vi "nanocal -- nuclear schottky fit V8.vi"() -> ()   [LabVIEW 2021] (continued)
\"σlogτS\" -> 0.000000000000   ,  \"σlogτN\" -> 0.000000000000   ,  \"σητ1\" -> 0.000000000000   ,  \"σητS \" -> 0.000000000000   ,  \"σητN\" -> 0.000000000000    |>   , \n\"IDS0571_220607_RAW_cal__ref_\" ->   <|    \"ζ\" -> 0.017026202892   ,  \"τ1\" -> 0.018855414009   ,  \"τS\" -> 0.047086117348   ,  \"τN\" -> 0.000023679327   ,  \"τC\" -> 0.002651600111   ,  \"κ0\" -> 0.000000012631   ,  \"mm1\" -> 0.000042096925   ,  \"mm2\" -> 0.018841082396   ,  \"mm3\" -> 0.050535732431   ,  \"T\" -> 1.900000000000   ,  \"B\" -> 2.000000000000   ,  \"θ\" -> 0.000000000000   ,  \"Reoff\" -> -457142.857142857042   ,  \"Imoff\" -> 0.000000000000   ,  \"στ1\" -> 0.700233981740   ,  \"στS\" -> 0.000265032226   ,  \"στN\" -> 0.457232881356   ,  \"τ11 \" -> 0.000000000000   ,  \"τ12\" -> 0.000000000000   ,  \"τ22\" -> 0.000000000000   ,  \"τN1\" -> 0.000000000000   ,  \"τN2\" -> 0.000000000000   ,  \"σηlogτ1 \" -> 0.000000000000   ,  \"σηlogτS\" -> 0.000000000000   ,  \"σηlogτN\" -> 0.000000000000   ,  \"σlogτ1\" -> 0.000000000000   ,  \"σlogτS\" -> 0.000000000000   ,  \"σlogτN\" -> 0.000000000000   ,  \"σητ1\" -> 0.000000000000   ,  \"σητS \" -> 0.000000000000   ,  \"σητN\" -> 0.000000000000    |>   , \n\"IDS0571_220607_RAW_cal__sam_\" ->   <|    \"ζ\" -> 0.000000000000   ,  \"τ1\" -> 0.000000000000   ,  \"τS\" -> 0.000000000000   ,  \"τN\" -> 0.000000000000   ,  \"τC\" -> 0.000000000000   ,  \"κ0\" -> 0.000000000000   ,  \"mm1\" -> 0.000000000000   ,  \"mm2\" -> 0.000000000000   ,  \"mm3\" -> 0.000000000000   ,  \"T\" -> 1.900000000000   ,  \"B\" -> 2.000000000000   ,  \"θ\" -> 0.000000000000   ,  \"Reoff\" -> 0.000000000000   ,  \"Imoff\" -> 0.000000000000   ,  \"στ1\" -> 0.000000000000   ,  \"στS\" -> 0.000000000000   ,  \"στN\" -> 0.000000000000   ,  \"τ11 \" -> 0.000000000000   ,  \"τ12\" -> 0.000000000000   ,  \"τ22\" -> 0.000000000000   ,  \"τN1\" -> 0.000000000000   ,  \"τN2\" -> 0.000000000000   ,  \"σηlogτ1 \" -> 0.000000000000   ,  \"σηlogτS\" -> 0.000000000000   ,  \"σηlogτN\" -> 0.000000000000   ,  \"σlogτ1\" -> 0.000000000000   ,  \"σlogτS\" -> 0.000000000000   ,  \"σlogτN\" -> 0.000000000000   ,  \"σητ1\" -> 0.000000000000   ,  \"σητS \" -> 0.000000000000   ,  \"σητN\" -> 0.000000000000    |>   , \n\"IDS0572_220607_RAW_cal__ref_\" ->   <|    \"ζ\" -> 0.018157472970   ,  \"τ1\" -> 0.020617918401   ,  \"τS\" -> 0.014016495736   ,  \"τN\" -> 0.000014742683   ,  \"τC\" -> 0.002574156451   ,  \"κ0\" -> 0.000000016091   ,  \"mm1\" -> 0.000038981702   ,  \"mm2\" -> 0.016741377131   ,  \"mm3\" -> 0.020697726271   ,  \"T\" -> 2.300000000000   ,  \"B\" -> 2.000000000000   ,  \"θ\" -> 0.000000000000   ,  \"Reoff\" -> -420408.163265306036   ,  \"Imoff\" -> 0.000000000000   ,  \"στ1\" -> 0.362521056079   ,  \"στS\" -> 0.000160694817   ,  \"στN\" -> 0.168025207283   ,  \"τ11 \" -> 0.000000000000   ,  \"τ12\" -> 0.000000000000   ,  \"τ22\" -> 0.000000000000   ,  \"τN1\" -> 0.000000000000   ,  \"τN2\" -> 0.000000000000   ,  \"σηlogτ1 \" -> 0.000000000000   ,  \"σηlogτS\" -> 0.000000000000   ,  \"σηlogτN\" -> 0.000000000000   ,  \"σlogτ1\" -> 0.000000000000   ,  \"σlogτS\" -> 0.000000000000   ,  \"σlogτN\" -> 0.000000000000   ,  \"σητ1\" -> 0.000000000000   ,  \"σητS \" -> 0.000000000000   ,  \"σητN\" -> 0.000000000000    |>   , \n\"IDS0572_220607_RAW_cal__sam_\" ->   <|    \"ζ\" -> 0.000000000000   ,  \"τ1\" -> 0.000000000000   ,  \"τS\" -> 0.000000000000   ,  \"τN\" -> 0.000000000000   ,  \"τC\" -> 0.000000000000   ,  \"κ0\" -> 0.000000000000   ,  \"mm1\" -> 0.000000000000   ,  \"mm2\" -> 0.000000000000   ,  \"mm3\" -> 0.000000000000   ,  \"T\" -> 2.300000000000   ,  \"B\" -> 2.000000000000   ,  \"θ\" -> 0.000000000000   ,  \"Reoff\" -> 0.000000000000   ,  \"Imoff\" -> 0.000000000000   ,  \"στ1\" -> 0.000000000000   ,  \"στS\" -> 0.000000000000   ,  \"στN\" -> 0.000000000000   ,  \"τ11 \" -> 0.000000000000   ,  \"τ12\" -> 0.000000000000   ,  \"τ22\" -> 0.000000000000   ,  \"τN1\" -> 0.000000000000   ,  \"τN2\" -> 0.000000000000   ,  \"σηlogτ1 \" -> 0.000000000000   ,  \"σηlogτS\" -> 0.000000000000   ,  \"σηlogτN\" -> 0.000000000000   ,  \"σlogτ1\" -> 0.000000000000   ,  \"σlogτS\" -> 0.000000000000   ,  \"σlogτN\" -> 0.000000000000   ,  \"σητ1\" -> 0.000000000000   ,  \"σητS \" -> 0.000000000000   ,  \"σητN\" -> 0.000000000000    |>   , \n\"IDS0573_220607_RAW_cal__ref_\" ->   <|    \"ζ\" -> 0.021415792037   ,  \"τ1\" -> 0.017082452868   ,  \"τS\" -> 0.009548586507   ,  \"τN\" -> 0.000007399205   ,  \"τC\" -> 0.002472586118   ,  \"κ0\" -> 0.000000022500   ,  \"mm1\" -> 0.000041498148   ,  \"mm2\" -> 0.012165481918   ,  \"mm3\" -> 0.017108693634   ,  \"T\" -> 3.100000000000   ,  \"B\" -> 2.000000000000   ,  \"θ\" -> 0.000000000000   ,  \"Reoff\" -> -261224.489795918343   ,  \"Imoff\" -> 0.000000000000   ,  \"στ1\" -> 0.720539777711   ,  \"στS\" -> 0.000216738961   ,  \"στN\" -> 0.337779672751   ,  \"τ11 \" -> 0.000000000000   ,  \"τ12\" -> 0.000000000000   ,  \"τ22\" -> 0.000000000000   ,  \"τN1\" -> 0.000000000000   ,  \"τN2\" -> 0.000000000000   ,  \"σηlogτ1 \" -> 0.000000000000   ,  \"σηlogτS\" -> 0.000000000000   ,  \"σηlogτN\" -> 0.000000000000   ,  \"σlogτ1\" -> 0.000000000000   ,  \"σlogτS\" -> 0.000000000000   ,  \"σlogτN\" -> 0.000000000000   ,  \"σητ1\" -> 0.000000000000   ,  \"σητS \" -> 0.000000000000   ,  \"σητN\" -> 0.000000000000    |>   , \n\"IDS0573_220607_RAW_cal__sam_\" ->   <|    \"ζ\" -> 0.000000000000   ,  \"τ1\" -> 0.000000000000   ,  \"τS\" -> 0.000000000000   ,  \"τN\" -> 0.000000000000   ,  \"τC\" -> 0.000000000000   ,  \"κ0\" -> 0.000000000000   ,  \"mm1\" -> 0.000000000000   ,  \"mm2\" -> 0.000000000000   ,  \"mm3\" -> 0.000000000000   ,  \"T\" -> 3.100000000000   ,  \"B\" -> 2.000000000000   ,  \"θ\" -> 0.000000000000   ,  \"Reoff\" -> 0.000000000000   ,  \"Imoff\" -> 0.000000000000   ,  \"στ1\" -> 0.000000000000   ,  \"στS\" -> 0.000000000000   ,  \"στN\" -> 0.000000000000   ,  \"τ11 \" -> 0.000000000000   ,  \"τ12\" -> 0.000000000000   ,  \"τ22\" -> 0.000000000000   ,  \"τN1\" -> 0.000000000000   ,  \"τN2\" -> 0.000000000000   ,  \"σηlogτ1 \" -> 0.000000000000   ,  \"σηlogτS\" -> 0.000000000000   ,  \"σηlogτN\" -> 0.000000000000   ,  \"σlogτ1\" -> 0.000000000000   ,  \"σlogτS\" -> 0.000000000000   ,  \"σlogτN\" -> 0.000000000000   ,  \"σητ1\" -> 0.000000000000   ,  \"σητS \" -> 0.000000000000   ,  \"σητN\" -> 0.000000000000    |>   , \n\"IDS0574_220607_RAW_cal__ref_\" ->   <|    \"ζ\" -> 0.022252360347   ,  \"τ1\" -> 0.015843819663   ,  \"τS\" -> 0.005763523322   ,  \"τN\" -> 0.000001375995   ,  \"τC\" -> 0.001974723590   ,  \"κ0\" -> 0.000000055533   ,  \"mm1\" -> 0.000032327889   ,  \"mm2\" -> 0.007832797575   ,  \"mm3\" -> 0.015846599723   ,  \"T\" -> 5.700000000000   ,  \"B\" -> 2.000000000000   ,  \"θ\" -> 0.000000000000   ,  \"Reoff\" -> -92244.897959183683   ,  \"Imoff\" -> 0.000000000000   ,  \"στ1\" -> 6.958139019645   ,  \"στS\" -> 0.000482683411   ,  \"στN\" -> 3.920374328535   ,  \"τ11 \" -> 0.000000000000   ,  \"τ12\" -> 0.000000000000   ,  \"τ22\" -> 0.000000000000   ,  \"τN1\" -> 0.000000000000   ,  \"τN2\" -> 0.000000000000   ,  \"σηlogτ1 \" -> 0.000000000000   ,  \"σηlogτS\" -> 0.000000000000   ,  \"σηlogτN\" -> 0.000000000000   ,  \"σlogτ1\" -> 0.000000000000   ,  \"σlogτS\" -> 0.000000000000   ,  \"σlogτN\" -> 0.000000000000   ,  \"σητ1\" -> 0.000000000000   ,  \"σητS \" -> 0.000000000000   ,  \"σητN\" -> 0.000000000000    |>   , \n\"IDS0574_220607_RAW_cal__sam_\" ->   <|    \"ζ\" -> 0.000000000000   ,  \"τ1\" -> 0.000000000000   ,  \"τS\" -> 0.000000000000   ,  \"τN\" -> 0.000000000000   ,  \"τC\" -> 0.000000000000   ,  \"κ0\" -> 0.000000000000   ,  \"mm1\" -> 0.000000000000   ,  \"mm2\" -> 0.000000000000   ,  \"mm3\" -> 0.000000000000   ,  \"T\" -> 5.700000000000   ,  \"B\" -> 2.000000000000   ,  \"θ\" -> 0.000000000000   ,  \"Reoff\" -> 0.000000000000   ,  \"Imoff\" -> 0.000000000000   ,  \"στ1\" -> 0.000000000000   ,  \"στS\" -> 0.000000000000   ,  \"στN\" -> 0.000000000000   ,  \"τ11 \" -> 0.000000000000   ,  \"τ12\" -> 0.000000000000   ,  \"τ22\" -> 0.000000000000   ,  \"τN1\" -> 0.000000000000   ,  \"τN2\" -> 0.000000000000   ,  \"σηlogτ1 \" -> 0.000000000000   ,  \"σηlogτS\" -> 0.000000000000   ,  \"σηlogτN\" -> 0.000000000000   ,  \"σlogτ1\" -> 0.000000000000   ,  \"σlogτS\" -> 0.000000000000   ,  \"σlogτN\" -> 0.000000000000   ,  \"σητ1\" -> 0.000000000000   ,  \"σητS \" -> 0.000000000000   ,  \"σητN\" -> 0.000000000000    |>   , \n\"IDS0578_220608_RAW_cal__ref_\" ->   <|    \"ζ\" -> 0.254942126755   ,  \"τ1\" -> 0.090194641149   ,  \"τS\" -> 0.019458727705   ,  \"τN\" -> 0.002319182302   ,  \"τC\" -> 0.000961097925   ,  \"κ0\" -> 0.000000000915   ,  \"mm1\" -> 0.000189263930   ,  \"mm2\" -> 0.024128719117   ,  \"mm3\" -> 0.094167772727   ,  \"T\" -> 0.200000000000   ,  \"B\" -> 2.000000000000   ,  \"θ\" -> 90.000000000000   ,  \"Reoff\" -> 0.000000000000   ,  \"Imoff\" -> 0.000000000000   ,  \"στ1\" -> 0.002629714713   ,  \"στS\" -> 0.000006197246   ,  \"στN\" -> 0.000056566732   ,  \"τ11 \" -> 0.000000000000   ,  \"τ12\" -> 0.000000000000   ,  \"τ22\" -> 0.000000000000   ,  \"τN1\" -> 0.000000000000   ,  \"τN2\" -> 0.000000000000   ,  \"σηlogτ1 \" -> 0.069428028467   ,  \"σηlogτS\" -> 0.000045157290   ,  \"σηlogτN\" -> 0.118005576339   ,  \"σlogτ1\" -> 0.029155997290   ,  \"σlogτS\" -> 0.000318481580   ,  \"σlogτN\" -> 0.024390808828   ,  \"σητ1\" -> 0.006262036113   ,  \"σητS \" -> 0.000000878703   ,  \"σητN\" -> 0.000273676444    |>   , \n\"IDS0578_220608_RAW_cal__sam_\" ->   <|    \"ζ\" -> 0.000000000000   ,  \"τ1\" -> 0.000000000000   ,  \"τS\" -> 0.000000000000   ,  \"τN\" -> 0.000000000000   ,  \"τC\" -> 0.000000000000   ,  \"κ0\" -> 0.000000000000   ,  \"mm1\" -> 0.000000000000   ,  \"mm2\" -> 0.000000000000   ,  \"mm3\" -> 0.000000000000   ,  \"T\" -> 0.200000000000   ,  \"B\" -> 2.000000000000   ,  \"θ\" -> 90.000000000000   ,  \"Reoff\" -> 0.000000000000   ,  \"Imoff\" -> 0.000000000000   ,  \"στ1\" -> 0.000000000000   ,  \"στS\" -> 0.000000000000   ,  \"στN\" -> 0.000000000000   ,  \"τ11 \" -> 0.000000000000   ,  \"τ12\" -> 0.000000000000   ,  \"τ22\" -> 0.000000000000   ,  \"τN1\" -> 0.000000000000   ,  \"τN2\" -> 0.000000000000   ,  \"σηlogτ1 \" -> 0.000000000000   ,  \"σηlogτS\" -> 0.000000000000   ,  \"σηlogτN\" -> 0.000000000000   ,  \"σlogτ1\" -> 0.000000000000   ,  \"σlogτS\" -> 0.000000000000   ,  \"σlogτN\" -> 0.000000000000   ,  \"σητ1\" -> 0.000000000000   ,  \"σητS \" -> 0.000000000000   ,  \"σητN\" -> 0.000000000000    |>   , \n\"IDS0579_220608_RAW_cal__ref_\" ->   <|    \"ζ\" -> 0.354589792209   ,  \"τ1\" -> 0.123845684439   ,  \"τS\" -> 0.022131661400   ,  \"τN\" -> 0.006759309931   ,  \"τC\" -> 0.000842117409   ,  \"κ0\" -> 0.000000000715   ,  \"mm1\" -> 0.000215927769   ,  \"mm2\" -> 0.027938681410   ,  \"mm3\" -> 0.135668607521   ,  \"T\" -> 0.170000000000   ,  \"B\" -> 2.000000000000   ,  \"θ\" -> 90.000000000000   ,  \"Reoff\" -> 0.000000000000   ,  \"Imoff\" -> 0.000000000000   ,  \"στ1\" -> 0.001777181665   ,  \"στS\" -> 0.000007534975   ,  \"στN\" -> 0.000083134209   ,  \"τ11 \" -> 0.000000000000   ,  \"τ12\" -> 0.000000000000   ,  \"τ22\" -> 0.000000000000   ,  \"τN1\" -> 0.000000000000   ,  \"τN2\" -> 0.000000000000   ,  \"σηlogτ1 \" -> 0.067674066824   ,  \"σηlogτS\" -> 0.000091288111   ,  \"σηlogτN\" -> 0.117525946822   ,  \"σlogτ1\" -> 0.014349968453   ,  \"σlogτS\" -> 0.000340461346   ,  \"σlogτN\" -> 0.012299215430   ,  \"σητ1\" -> 0.008381141125   ,  \"σητS \" -> 0.000002020358   ,  \"σητN\" -> 0.000794394299    |>   , \n\"IDS0579_220608_RAW_cal__sam_\" ->   <|    \"ζ\" -> 0.000000000000   ,  \"τ1\" -> 0.000000000000   ,  \"τS\" -> 0.000000000000   ,  \"τN\" -> 0.000000000000   ,  \"τC\" -> 0.000000000000   ,  \"κ0\" -> 0.000000000000   ,  \"mm1\" -> 0.000000000000   ,  \"mm2\" -> 0.000000000000   ,  \"mm3\" -> 0.000000000000   ,  \"T\" -> 0.170000000000   ,  \"B\" -> 2.000000000000   ,  \"θ\" -> 90.000000000000   ,  \"Reoff\" -> 0.000000000000   ,  \"Imoff\" -> 0.000000000000   ,  \"στ1\" -> 0.000000000000   ,  \"στS\" -> 0.000000000000   ,  \"στN\" -> 0.000000000000   ,  \"τ11 \" -> 0.000000000000   ,  \"τ12\" -> 0.000000000000   ,  \"τ22\" -> 0.000000000000   ,  \"τN1\" -> 0.000000000000   ,  \"τN2\" -> 0.000000000000   ,  \"σηlogτ1 \" -> 0.000000000000   ,  \"σηlogτS\" -> 0.000000000000   ,  \"σηlogτN\" -> 0.000000000000   ,  \"σlogτ1\" -> 0.000000000000   ,  \"σlogτS\" -> 0.000000000000   ,  \"σlogτN\" -> 0.000000000000   ,  \"σητ1\" -> 0.000000000000   ,  \"σητS \" -> 0.000000000000   ,  \"σητN\" -> 0.000000000000    |>   , \n\"IDS0580_220608_RAW_cal__ref_\" ->   <|    \"ζ\" -> 0.444346939390   ,  \"τ1\" -> 0.140421584261   ,  \"τS\" -> 0.025124829385   ,  \"τN\" -> 0.007555288626   ,  \"τC\" -> 0.000880068073   ,  \"κ0\" -> 0.000000000613   ,  \"mm1\" -> 0.000266242992   ,  \"mm2\" -> 0.033486096652   ,  \"mm3\" -> 0.154750741118   ,  \"T\" -> 0.150000000000   ,  \"B\" -> 2.000000000000   ,  \"θ\" -> 90.000000000000   ,  \"Reoff\" -> 0.000000000000   ,  \"Imoff\" -> 0.000000000000   ,  \"στ1\" -> 0.003309353978   ,  \"στS\" -> 0.000014809905   ,  \"στN\" -> 0.000151067842   ,  \"τ11 \" -> 0.000000000000   ,  \"τ12\" -> 0.000000000000   ,  \"τ22\" -> 0.000000000000   ,  \"τN1\" -> 0.000000000000   ,  \"τN2\" -> 0.000000000000   ,  \"σηlogτ1 \" -> 0.068601733004   ,  \"σηlogτS\" -> 0.000100884728   ,  \"σηlogτN\" -> 0.117829477099   ,  \"σlogτ1\" -> 0.023567274184   ,  \"σlogτS\" -> 0.000589452965   ,  \"σlogτN\" -> 0.019994979637   ,  \"σητ1\" -> 0.009633164031   ,  \"σητS \" -> 0.000002534712   ,  \"σητN\" -> 0.000890235708    |>   , \n\"IDS0580_220608_RAW_cal__sam_\" ->   <|    \"ζ\" -> 0.000000000000   ,  \"τ1\" -> 0.000000000000   ,  \"τS\" -> 0.000000000000   ,  \"τN\" -> 0.000000000000   ,  \"τC\" -> 0.000000000000   ,  \"κ0\" -> 0.000000000000   ,  \"mm1\" -> 0.000000000000   ,  \"mm2\" -> 0.000000000000   ,  \"mm3\" -> 0.000000000000   ,  \"T\" -> 0.150000000000   ,  \"B\" -> 2.000000000000   ,  \"θ\" -> 90.000000000000   ,  \"Reoff\" -> 0.000000000000   ,  \"Imoff\" -> 0.000000000000   ,  \"στ1\" -> 0.000000000000   ,  \"στS\" -> 0.000000000000   ,  \"στN\" -> 0.000000000000   ,  \"τ11 \" -> 0.000000000000   ,  \"τ12\" -> 0.000000000000   ,  \"τ22\" -> 0.000000000000   ,  \"τN1\" -> 0.000000000000   ,  \"τN2\" -> 0.000000000000   ,  \"σηlogτ1 \" -> 0.000000000000   ,  \"σηlogτS\" -> 0.000000000000   ,  \"σηlogτN\" -> 0.000000000000   ,  \"σlogτ1\" -> 0.000000000000   ,  \"σlogτS\" -> 0.000000000000   ,  \"σlogτN\" -> 0.000000000000   ,  \"σητ1\" -> 0.000000000000   ,  \"σητS \" -> 0.000000000000   ,  \"σητN\" -> 0.000000000000    |>   , \n\"IDS0581_220608_RAW_cal__ref_\" ->   <|    \"ζ\" -> 0.655027140715   ,  \"τ1\" -> 0.183223097165   ,  \"τS\" -> 0.032562109692   ,  \"τN\" -> 0.027297213493   ,  \"τC\" -> 0.000898478349   ,  \"κ0\" -> 0.000000000448   ,  \"mm1\" -> 0.000352024750   ,  \"mm2\" -> 0.041294300607   ,  \"mm3\" -> 0.241544054651   ,  \"T\" -> 0.120000000000   ,  \"B\" -> 2.000000000000   ,  \"θ\" -> 90.000000000000   ,  \"Reoff\" -> 0.000000000000   ,  \"Imoff\" -> 0.000000000000   ,  \"στ1\" -> 0.001245243248   ,  \"στS\" -> 0.000016061611   ,  \"στN\" -> 0.000155520175   ,  \"τ11 \" -> 0.000000000000   ,  \"τ12\" -> 0.000000000000   ,  \"τ22\" -> 0.000000000000   ,  \"τN1\" -> 0.000000000000   ,  \"τN2\" -> 0.000000000000   ,  \"σηlogτ1 \" -> 0.071224317656   ,  \"σηlogτS\" -> 0.000341404704   ,  \"σηlogτN\" -> 0.119101614664   ,  \"σlogτ1\" -> 0.006796322447   ,  \"σlogτS\" -> 0.000493260767   ,  \"σlogτN\" -> 0.005697291241   ,  \"σητ1\" -> 0.013049940074   ,  \"σητS \" -> 0.000011116857   ,  \"σητN\" -> 0.003251142203    |>   , \n\"IDS0581_220608_RAW_cal__sam_\" ->   <|    \"ζ\" -> 0.000000000000   ,  \"τ1\" -> 0.000000000000   ,  \"τS\" -> 0.000000000000   ,  \"τN\" -> 0.000000000000   ,  \"τC\" -> 0.000000000000   ,  \"κ0\" -> 0.000000000000   ,  \"mm1\" -> 0.000000000000   ,  \"mm2\" -> 0.000000000000   ,  \"mm3\" -> 0.000000000000   ,  \"T\" -> 0.120000000000   ,  \"B\" -> 2.000000000000   ,  \"θ\" -> 90.000000000000   ,  \"Reoff\" -> 0.000000000000   ,  \"Imoff\" -> 0.000000000000   ,  \"στ1\" -> 0.000000000000   ,  \"στS\" -> 0.000000000000   ,  \"στN\" -> 0.000000000000   ,  \"τ11 \" -> 0.000000000000   ,  \"τ12\" -> 0.000000000000   ,  \"τ22\" -> 0.000000000000   ,  \"τN1\" -> 0.000000000000   ,  \"τN2\" -> 0.000000000000   ,  \"σηlogτ1 \" -> 0.000000000000   ,  \"σηlogτS\" -> 0.000000000000   ,  \"σηlogτN\" -> 0.000000000000   ,  \"σlogτ1\" -> 0.000000000000   ,  \"σlogτS\" -> 0.000000000000   ,  \"σlogτN\" -> 0.000000000000   ,  \"σητ1\" -> 0.000000000000   ,  \"σητS \" -> 0.000000000000   ,  \"σητN\" -> 0.000000000000    |>   , \n\"IDS0582_220608_RAW_cal__ref_\" ->   <|    \"ζ\" -> 0.162998508749   ,  \"τ1\" -> 0.143783108641   ,  \"τS\" -> 0.016635646203   ,  \"τN\" -> 0.002767018248   ,  \"τC\" -> 0.001004852281   ,  \"κ0\" -> 0.000000001234   ,  \"mm1\" -> 0.000134771852   ,  \"mm2\" -> 0.019706367751   ,  \"mm3\" -> 0.147512091141   ,  \"T\" -> 0.250000000000   ,  \"B\" -> 2.000000000000   ,  \"θ\" -> 90.000000000000   ,  \"Reoff\" -> 0.000000000000   ,  \"Imoff\" -> 0.000000000000   ,  \"στ1\" -> 0.002611343542   ,  \"στS\" -> 0.000002038066   ,  \"στN\" -> 0.000046147830   ,  \"τ11 \" -> 0.000000000000   ,  \"τ12\" -> 0.000000000000   ,  \"τ22\" -> 0.000000000000   ,  \"τN1\" -> 0.000000000000   ,  \"τN2\" -> 0.000000000000   ,  \"σηlogτ1 \" -> 0.061276541493   ,  \"σηlogτS\" -> 0.000016947124   ,  \"σηlogτN\" -> 0.115361584710   ,  \"σlogτ1\" -> 0.018161685100   ,  \"σlogτS\" -> 0.000122511986   ,  \"σlogτN\" -> 0.016677819318   ,  \"σητ1\" -> 0.008810531623   ,  \"σητS \" -> 0.000000281926   ,  \"σητN\" -> 0.000319207610    |>   , \n\"IDS0582_220608_RAW_cal__sam_\" ->   <|    \"ζ\" -> 0.000000000000   ,  \"τ1\" -> 0.000000000000   ,  \"τS\" -> 0.000000000000   ,  \"τN\" -> 0.000000000000   ,  \"τC\" -> 0.000000000000   ,  \"κ0\" -> 0.000000000000   ,  \"mm1\" -> 0.000000000000   ,  \"mm2\" -> 0.000000000000   ,  \"mm3\" -> 0.000000000000   ,  \"T\" -> 0.250000000000   ,  \"B\" -> 2.000000000000   ,  \"θ\" -> 90.000000000000   ,  \"Reoff\" -> 0.000000000000   ,  \"Imoff\" -> 0.000000000000   ,  \"στ1\" -> 0.000000000000   ,  \"στS\" -> 0.000000000000   ,  \"στN\" -> 0.000000000000   ,  \"τ11 \" -> 0.000000000000   ,  \"τ12\" -> 0.000000000000   ,  \"τ22\" -> 0.000000000000   ,  \"τN1\" -> 0.000000000000   ,  \"τN2\" -> 0.000000000000   ,  \"σηlogτ1 \" -> 0.000000000000   ,  \"σηlogτS\" -> 0.000000000000   ,  \"σηlogτN\" -> 0.000000000000   ,  \"σlogτ1\" -> 0.000000000000   ,  \"σlogτS\" -> 0.000000000000   ,  \"σlogτN\" -> 0.000000000000   ,  \"σητ1\" -> 0.000000000000   ,  \"σητS \" -> 0.000000000000   ,  \"σητN\" -> 0.000000000000    |>   , \n\"IDS0583_220608_RAW_cal__ref_\" ->   <|    \"ζ\" -> 0.113859081836   ,  \"τ1\" -> 0.043737196942   ,  \"τS\" -> 0.015314148754   ,  \"τN\" -> 0.001020465976   ,  \"τC\" -> 0.001208611456   ,  \"κ0\" -> 0.000000001554   ,  \"mm1\" -> 0.000116107054   ,  \"mm2\" -> 0.017399705428   ,  \"mm3\" -> 0.045624454882   ,  \"T\" -> 0.300000000000   ,  \"B\" -> 2.000000000000   ,  \"θ\" -> 90.000000000000   ,  \"Reoff\" -> 0.000000000000   ,  \"Imoff\" -> 0.000000000000   ,  \"στ1\" -> 0.000581466774   ,  \"στS\" -> 0.000001888292   ,  \"στN\" -> 0.000010385640   ,  \"τ11 \" -> 0.000000000000   ,  \"τ12\" -> 0.000000000000   ,  \"τ22\" -> 0.000000000000   ,  \"τN1\" -> 0.000000000000   ,  \"τN2\" -> 0.000000000000   ,  \"σηlogτ1 \" -> 0.077320715049   ,  \"σηlogτS\" -> 0.000052774422   ,  \"σηlogτN\" -> 0.120352981803   ,  \"σlogτ1\" -> 0.013294559654   ,  \"σlogτS\" -> 0.000123303775   ,  \"σlogτN\" -> 0.010177350905   ,  \"σητ1\" -> 0.003381791342   ,  \"σητS \" -> 0.000000808195   ,  \"σητN\" -> 0.000122816123    |>   , \n\"IDS0583_220608_RAW_cal__sam_\" ->   <|    \"ζ\" -> 0.000000000000   ,  \"τ1\" -> 0.000000000000   ,  \"τS\" -> 0.000000000000   ,  \"τN\" -> 0.000000000000   ,  \"τC\" -> 0.000000000000   ,  \"κ0\" -> 0.000000000000   ,  \"mm1\" -> 0.000000000000   ,  \"mm2\" -> 0.000000000000   ,  \"mm3\" -> 0.000000000000   ,  \"T\" -> 0.300000000000   ,  \"B\" -> 2.000000000000   ,  \"θ\" -> 90.000000000000   ,  \"Reoff\" -> 0.000000000000   ,  \"Imoff\" -> 0.000000000000   ,  \"στ1\" -> 0.000000000000   ,  \"στS\" -> 0.000000000000   ,  \"στN\" -> 0.000000000000   ,  \"τ11 \" -> 0.000000000000   ,  \"τ12\" -> 0.000000000000   ,  \"τ22\" -> 0.000000000000   ,  \"τN1\" -> 0.000000000000   ,  \"τN2\" -> 0.000000000000   ,  \"σηlogτ1 \" -> 0.000000000000   ,  \"σηlogτS\" -> 0.000000000000   ,  \"σηlogτN\" -> 0.000000000000   ,  \"σlogτ1\" -> 0.000000000000   ,  \"σlogτS\" -> 0.000000000000   ,  \"σlogτN\" -> 0.000000000000   ,  \"σητ1\" -> 0.000000000000   ,  \"σητS \" -> 0.000000000000   ,  \"σητN\" -> 0.000000000000    |>   , \n\"IDS0584_220608_RAW_cal__ref_\" ->   <|    \"ζ\" -> 0.081243214747   ,  \"τ1\" -> 0.037135443189   ,  \"τS\" -> 0.014363776862   ,  \"τN\" -> 0.000724531165   ,  \"τC\" -> 0.001657389357   ,  \"κ0\" -> 0.000000001966   ,  \"mm1\" -> 0.000113270602   ,  \"mm2\" -> 0.016452146337   ,  \"mm3\" -> 0.038541546284   ,  \"T\" -> 0.360000000000   ,  \"B\" -> 2.000000000000   ,  \"θ\" -> 90.000000000000   ,  \"Reoff\" -> 0.000000000000   ,  \"Imoff\" -> 0.000000000000   ,  \"στ1\" -> 0.000570634052   ,  \"στS\" -> 0.000001716733   ,  \"στN\" -> 0.000008284109   ,  \"τ11 \" -> 0.000000000000   ,  \"τ12\" -> 0.000000000000   ,  \"τ22\" -> 0.000000000000   ,  \"τN1\" -> 0.000000000000   ,  \"τN2\" -> 0.000000000000   ,  \"σηlogτ1 \" -> 0.079922172346   ,  \"σηlogτS\" -> 0.000048378934   ,  \"σηlogτN\" -> 0.121081817682   ,  \"σlogτ1\" -> 0.015366291700   ,  \"σlogτS\" -> 0.000119518229   ,  \"σlogτN\" -> 0.011433750926   ,  \"σητ1\" -> 0.002967945291   ,  \"σητS \" -> 0.000000694904   ,  \"σητN\" -> 0.000087727550    |>   , \n\"IDS0584_220608_RAW_cal__sam_\" ->   <|    \"ζ\" -> 0.000000000000   ,  \"τ1\" -> 0.000000000000   ,  \"τS\" -> 0.000000000000   ,  \"τN\" -> 0.000000000000   ,  \"τC\" -> 0.000000000000   ,  \"κ0\" -> 0.000000000000   ,  \"mm1\" -> 0.000000000000   ,  \"mm2\" -> 0.000000000000   ,  \"mm3\" -> 0.000000000000   ,  \"T\" -> 0.360000000000   ,  \"B\" -> 2.000000000000   ,  \"θ\" -> 90.000000000000   ,  \"Reoff\" -> 0.000000000000   ,  \"Imoff\" -> 0.000000000000   ,  \"στ1\" -> 0.000000000000   ,  \"στS\" -> 0.000000000000   ,  \"στN\" -> 0.000000000000   ,  \"τ11 \" -> 0.000000000000   ,  \"τ12\" -> 0.000000000000   ,  \"τ22\" -> 0.000000000000   ,  \"τN1\" -> 0.000000000000   ,  \"τN2\" -> 0.000000000000   ,  \"σηlogτ1 \" -> 0.000000000000   ,  \"σηlogτS\" -> 0.000000000000   ,  \"σηlogτN\" -> 0.000000000000   ,  \"σlogτ1\" -> 0.000000000000   ,  \"σlogτS\" -> 0.000000000000   ,  \"σlogτN\" -> 0.000000000000   ,  \"σητ1\" -> 0.000000000000   ,  \"σητS \" -> 0.000000000000   ,  \"σητN\" -> 0.000000000000    |>   , \n\"IDS0585_220608_RAW_cal__ref_\" ->   <|    \"ζ\" -> 0.062678864922   ,  \"τ1\" -> 0.031193965489   ,  \"τS\" -> 0.014071158439   ,  \"τN\" -> 0.000589761795   ,  \"τC\" -> 0.002071432088   ,  \"κ0\" -> 0.000000002372   ,  \"mm1\" -> 0.000107994659   ,  \"mm2\" -> 0.016236809619   ,  \"mm3\" -> 0.032500443370   ,  \"T\" -> 0.420000000000   ,  \"B\" -> 2.000000000000   ,  \"θ\" -> 90.000000000000   ,  \"Reoff\" -> 0.000000000000   ,  \"Imoff\" -> 0.000000000000   ,  \"στ1\" -> 0.000397411460   ,  \"στS\" -> 0.000001349493   ,  \"στN\" -> 0.000005324437   ,  \"τ11 \" -> 0.000000000000   ,  \"τ12\" -> 0.000000000000   ,  \"τ22\" -> 0.000000000000   ,  \"τN1\" -> 0.000000000000   ,  \"τN2\" -> 0.000000000000   ,  \"σηlogτ1 \" -> 0.084702441661   ,  \"σηlogτS\" -> 0.000054291410   ,  \"σηlogτN\" -> 0.122395661985   ,  \"σlogτ1\" -> 0.012740010877   ,  \"σlogτS\" -> 0.000095904870   ,  \"σlogτN\" -> 0.009028114419   ,  \"σητ1\" -> 0.002642205042   ,  \"σητS \" -> 0.000000763943   ,  \"σητN\" -> 0.000072184285    |>   , \n\"IDS0585_220608_RAW_cal__sam_\" ->   <|    \"ζ\" -> 0.000000000000   ,  \"τ1\" -> 0.000000000000   ,  \"τS\" -> 0.000000000000   ,  \"τN\" -> 0.000000000000   ,  \"τC\" -> 0.000000000000   ,  \"κ0\" -> 0.000000000000   ,  \"mm1\" -> 0.000000000000   ,  \"mm2\" -> 0.000000000000   ,  \"mm3\" -> 0.000000000000   ,  \"T\" -> 0.420000000000   ,  \"B\" -> 2.000000000000   ,  \"θ\" -> 90.000000000000   ,  \"Reoff\" -> 0.000000000000   ,  \"Imoff\" -> 0.000000000000   ,  \"στ1\" -> 0.000000000000   ,  \"στS\" -> 0.000000000000   ,  \"στN\" -> 0.000000000000   ,  \"τ11 \" -> 0.000000000000   ,  \"τ12\" -> 0.000000000000   ,  \"τ22\" -> 0.000000000000   ,  \"τN1\" -> 0.000000000000   ,  \"τN2\" -> 0.000000000000   ,  \"σηlogτ1 \" -> 0.000000000000   ,  \"σηlogτS\" -> 0.000000000000   ,  \"σηlogτN\" -> 0.000000000000   ,  \"σlogτ1\" -> 0.000000000000   ,  \"σlogτS\" -> 0.000000000000   ,  \"σlogτN\" -> 0.000000000000   ,  \"σητ1\" -> 0.000000000000   ,  \"σητS \" -> 0.000000000000   ,  \"σητN\" -> 0.000000000000    |>   , \n\"IDS0586_220608_RAW_cal__ref_\" ->   <|    \"ζ\" -> 0.045613371440   ,  \"τ1\" -> 0.021724714281   ,  \"τS\" -> 0.014809258132   ,  \"τN\" -> 0.000242258752   ,  \"τC\" -> 0.002279252740   ,  \"κ0\" -> 0.000000003040   ,  \"mm1\" -> 0.000087097961   ,  \"mm2\" -> 0.016810935074   ,  \"mm3\" -> 0.022844001301   ,  \"T\" -> 0.520000000000   ,  \"B\" -> 2.000000000000   ,  \"θ\" -> 90.000000000000   ,  \"Reoff\" -> 0.000000000000   ,  \"Imoff\" -> 0.000000000000   ,  \"στ1\" -> 0.000379951004   ,  \"στS\" -> 0.000001062979   ,  \"στN\" -> 0.000002619514   ,  \"τ11 \" -> 0.000000000000   ,  \"τ12\" -> 0.000000000000   ,  \"τ22\" -> 0.000000000000   ,  \"τN1\" -> 0.000000000000   ,  \"τN2\" -> 0.000000000000   ,  \"σηlogτ1 \" -> 0.100214341065   ,  \"σηlogτS\" -> 0.000043367653   ,  \"σηlogτN\" -> 0.126292121784   ,  \"σlogτ1\" -> 0.017489344108   ,  \"σlogτS\" -> 0.000071778006   ,  \"σlogτN\" -> 0.010812876419   ,  \"σητ1\" -> 0.002177127926   ,  \"σητS \" -> 0.000000642243   ,  \"σητN\" -> 0.000030595372    |>   , \n\"IDS0586_220608_RAW_cal__sam_\" ->   <|    \"ζ\" -> 0.000000000000   ,  \"τ1\" -> 0.000000000000   ,  \"τS\" -> 0.000000000000   ,  \"τN\" -> 0.000000000000   ,  \"τC\" -> 0.000000000000   ,  \"κ0\" -> 0.000000000000   ,  \"mm1\" -> 0.000000000000   ,  \"mm2\" -> 0.000000000000   ,  \"mm3\" -> 0.000000000000   ,  \"T\" -> 0.520000000000   ,  \"B\" -> 2.000000000000   ,  \"θ\" -> 90.000000000000   ,  \"Reoff\" -> 0.000000000000   ,  \"Imoff\" -> 0.000000000000   ,  \"στ1\" -> 0.000000000000   ,  \"στS\" -> 0.000000000000   ,  \"στN\" -> 0.000000000000   ,  \"τ11 \" -> 0.000000000000   ,  \"τ12\" -> 0.000000000000   ,  \"τ22\" -> 0.000000000000   ,  \"τN1\" -> 0.000000000000   ,  \"τN2\" -> 0.000000000000   ,  \"σηlogτ1 \" -> 0.000000000000   ,  \"σηlogτS\" -> 0.000000000000   ,  \"σηlogτN\" -> 0.000000000000   ,  \"σlogτ1\" -> 0.000000000000   ,  \"σlogτS\" -> 0.000000000000   ,  \"σlogτN\" -> 0.000000000000   ,  \"σητ1\" -> 0.000000000000   ,  \"σητS \" -> 0.000000000000   ,  \"σητN\" -> 0.000000000000    |>   , \n\"IDS0587_220608_RAW_cal__ref_\" ->   <|    \"ζ\" -> 0.037305312817   ,  \"τ1\" -> 0.022015385532   ,  \"τS\" -> 0.015983002513   ,  \"τN\" -> 0.000140757523   ,  \"τC\" -> 0.002926821930   ,  \"κ0\" -> 0.000000003719   ,  \"mm1\" -> 0.000089879141   ,  \"mm2\" -> 0.018616997914   ,  \"mm3\" -> 0.022960592355   ,  \"T\" -> 0.620000000000   ,  \"B\" -> 2.000000000000   ,  \"θ\" -> 90.000000000000   ,  \"Reoff\" -> 0.000000000000   ,  \"Imoff\" -> 0.000000000000   ,  \"στ1\" -> 0.001387023615   ,  \"στS\" -> 0.000002362873   ,  \"στN\" -> 0.000005327242   ,  \"τ11 \" -> 0.000000000000   ,  \"τ12\" -> 0.000000000000   ,  \"τ22\" -> 0.000000000000   ,  \"τN1\" -> 0.000000000000   ,  \"τN2\" -> 0.000000000000   ,  \"σηlogτ1 \" -> 0.104062754618   ,  \"σηlogτS\" -> 0.000026827334   ,  \"σηlogτN\" -> 0.127171087311   ,  \"σlogτ1\" -> 0.063002467668   ,  \"σlogτS\" -> 0.000147836639   ,  \"σlogτN\" -> 0.037846942559   ,  \"σητ1\" -> 0.002290981662   ,  \"σητS \" -> 0.000000428781   ,  \"σητN\" -> 0.000017900287    |>   , \n\"IDS0587_220608_RAW_cal__sam_\" ->   <|    \"ζ\" -> 0.000000000000   ,  \"τ1\" -> 0.000000000000   ,  \"τS\" -> 0.000000000000   ,  \"τN\" -> 0.000000000000   ,  \"τC\" -> 0.000000000000   ,  \"κ0\" -> 0.000000000000   ,  \"mm1\" -> 0.000000000000   ,  \"mm2\" -> 0.000000000000   ,  \"mm3\" -> 0.000000000000   ,  \"T\" -> 0.620000000000   ,  \"B\" -> 2.000000000000   ,  \"θ\" -> 90.000000000000   ,  \"Reoff\" -> 0.000000000000   ,  \"Imoff\" -> 0.000000000000   ,  \"στ1\" -> 0.000000000000   ,  \"στS\" -> 0.000000000000   ,  \"στN\" -> 0.000000000000   ,  \"τ11 \" -> 0.000000000000   ,  \"τ12\" -> 0.000000000000   ,  \"τ22\" -> 0.000000000000   ,  \"τN1\" -> 0.000000000000   ,  \"τN2\" -> 0.000000000000   ,  \"σηlogτ1 \" -> 0.000000000000   ,  \"σηlogτS\" -> 0.000000000000   ,  \"σηlogτN\" -> 0.000000000000   ,  \"σlogτ1\" -> 0.000000000000   ,  \"σlogτS\" -> 0.000000000000   ,  \"σlogτN\" -> 0.000000000000   ,  \"σητ1\" -> 0.000000000000   ,  \"σητS \" -> 0.000000000000   ,  \"σητN\" -> 0.000000000000    |>   , \n\"IDS0588_220608_RAW_cal__ref_\" ->   <|    \"ζ\" -> 0.025909739103   ,  \"τ1\" -> 0.011339568662   ,  \"τS\" -> 0.019465034891   ,  \"τN\" -> 0.000064248096   ,  \"τC\" -> 0.003634951458   ,  \"κ0\" -> 0.000000005097   ,  \"mm1\" -> 0.000077921965   ,  \"mm2\" -> 0.011278943418   ,  \"mm3\" -> 0.023652936351   ,  \"T\" -> 0.820000000000   ,  \"B\" -> 2.000000000000   ,  \"θ\" -> 90.000000000000   ,  \"Reoff\" -> 0.000000000000   ,  \"Imoff\" -> 0.000000000000   ,  \"στ1\" -> 0.000804918682   ,  \"στS\" -> 0.000001968832   ,  \"στN\" -> 0.000002244062   ,  \"τ11 \" -> 0.000000000000   ,  \"τ12\" -> 0.000000000000   ,  \"τ22\" -> 0.000000000000   ,  \"τN1\" -> 0.000000000000   ,  \"τN2\" -> 0.000000000000   ,  \"σηlogτ1 \" -> 0.166612292303   ,  \"σηlogτS\" -> 0.000038744835   ,  \"σηlogτN\" -> 0.138837522658   ,  \"σlogτ1\" -> 0.070983183376   ,  \"σlogτS\" -> 0.000101147100   ,  \"σlogτN\" -> 0.034928067640   ,  \"σητ1\" -> 0.001889311528   ,  \"σητS \" -> 0.000000754170   ,  \"σητN\" -> 0.000008920046    |>   , \n\"IDS0588_220608_RAW_cal__sam_\" ->   <|    \"ζ\" -> 0.000000000000   ,  \"τ1\" -> 0.000000000000   ,  \"τS\" -> 0.000000000000   ,  \"τN\" -> 0.000000000000   ,  \"τC\" -> 0.000000000000   ,  \"κ0\" -> 0.000000000000   ,  \"mm1\" -> 0.000000000000   ,  \"mm2\" -> 0.000000000000   ,  \"mm3\" -> 0.000000000000   ,  \"T\" -> 0.820000000000   ,  \"B\" -> 2.000000000000   ,  \"θ\" -> 90.000000000000   ,  \"Reoff\" -> 0.000000000000   ,  \"Imoff\" -> 0.000000000000   ,  \"στ1\" -> 0.000000000000   ,  \"στS\" -> 0.000000000000   ,  \"στN\" -> 0.000000000000   ,  \"τ11 \" -> 0.000000000000   ,  \"τ12\" -> 0.000000000000   ,  \"τ22\" -> 0.000000000000   ,  \"τN1\" -> 0.000000000000   ,  \"τN2\" -> 0.000000000000   ,  \"σηlogτ1 \" -> 0.000000000000   ,  \"σηlogτS\" -> 0.000000000000   ,  \"σηlogτN\" -> 0.000000000000   ,  \"σlogτ1\" -> 0.000000000000   ,  \"σlogτS\" -> 0.000000000000   ,  \"σlogτN\" -> 0.000000000000   ,  \"σητ1\" -> 0.000000000000   ,  \"σητS \" -> 0.000000000000   ,  \"σητN\" -> 0.000000000000    |>   , \n\"IDS0589_220608_RAW_cal__ref_\" ->   <|    \"ζ\" -> 0.019947361770   ,  \"τ1\" -> 0.011361864478   ,  \"τS\" -> 0.027583078448   ,  \"τN\" -> 0.000020419433   ,  \"τC\" -> 0.003703000671   ,  \"κ0\" -> 0.000000007195   ,  \"mm1\" -> 0.000064126126   ,  \"mm2\" -> 0.011350297658   ,  \"mm3\" -> 0.031804556204   ,  \"T\" -> 1.120000000000   ,  \"B\" -> 2.000000000000   ,  \"θ\" -> 90.000000000000   ,  \"Reoff\" -> 0.000000000000   ,  \"Imoff\" -> 0.000000000000   ,  \"στ1\" -> 0.003857512169   ,  \"στS\" -> 0.000003346779   ,  \"στN\" -> 0.000003441616   ,  \"τ11 \" -> 0.000000000000   ,  \"τ12\" -> 0.000000000000   ,  \"τ22\" -> 0.000000000000   ,  \"τN1\" -> 0.000000000000   ,  \"τN2\" -> 0.000000000000   ,  \"σηlogτ1 \" -> 0.199481573795   ,  \"σηlogτS\" -> 0.000012934123   ,  \"σηlogτN\" -> 0.143434929162   ,  \"σlogτ1\" -> 0.339514009879   ,  \"σlogτS\" -> 0.000121334492   ,  \"σlogτN\" -> 0.168546132727   ,  \"σητ1\" -> 0.002266482607   ,  \"σητS \" -> 0.000000356763   ,  \"σητN\" -> 0.000002928860    |>   , \n\"IDS0589_220608_RAW_cal__sam_\" ->   <|    \"ζ\" -> 0.000000000000   ,  \"τ1\" -> 0.000000000000   ,  \"τS\" -> 0.000000000000   ,  \"τN\" -> 0.000000000000   ,  \"τC\" -> 0.000000000000   ,  \"κ0\" -> 0.000000000000   ,  \"mm1\" -> 0.000000000000   ,  \"mm2\" -> 0.000000000000   ,  \"mm3\" -> 0.000000000000   ,  \"T\" -> 1.120000000000   ,  \"B\" -> 2.000000000000   ,  \"θ\" -> 90.000000000000   ,  \"Reoff\" -> 0.000000000000   ,  \"Imoff\" -> 0.000000000000   ,  \"στ1\" -> 0.000000000000   ,  \"στS\" -> 0.000000000000   ,  \"στN\" -> 0.000000000000   ,  \"τ11 \" -> 0.000000000000   ,  \"τ12\" -> 0.000000000000   ,  \"τ22\" -> 0.000000000000   ,  \"τN1\" -> 0.000000000000   ,  \"τN2\" -> 0.000000000000   ,  \"σηlogτ1 \" -> 0.000000000000   ,  \"σηlogτS\" -> 0.000000000000   ,  \"σηlogτN\" -> 0.000000000000   ,  \"σlogτ1\" -> 0.000000000000   ,  \"σlogτS\" -> 0.000000000000   ,  \"σlogτN\" -> 0.000000000000   ,  \"σητ1\" -> 0.000000000000   ,  \"σητS \" -> 0.000000000000   ,  \"σητN\" -> 0.000000000000    |>   , \n\"IDS0590_220608_RAW_cal__ref_\" ->   <|    \"ζ\" -> 0.015986824181   ,  \"τ1\" -> 0.008744331225   ,  \"τS\" -> 0.042647705878   ,  \"τN\" -> 0.000007777315   ,  \"τC\" -> 0.003875042779   ,  \"κ0\" -> 0.000000010497   ,  \"mm1\" -> 0.000056035896   ,  \"mm2\" -> 0.008742533558   ,  \"mm3\" -> 0.047158213452   ,  \"T\" -> 1.600000000000   ,  \"B\" -> 2.000000000000   ,  \"θ\" -> 90.000000000000   ,  \"Reoff\" -> 0.000000000000   ,  \"Imoff\" -> 0.000000000000   ,  \"στ1\" -> 0.012923457313   ,  \"στS\" -> 0.000006598601   ,  \"στN\" -> 0.000006323440   ,  \"τ11 \" -> 0.000000000000   ,  \"τ12\" -> 0.000000000000   ,  \"τ22\" -> 0.000000000000   ,  \"τN1\" -> 0.000000000000   ,  \"τN2\" -> 0.000000000000   ,  \"σηlogτ1 \" -> 0.292115286414   ,  \"σηlogτS\" -> 0.000006686874   ,  \"σηlogτN\" -> 0.152613381435   ,  \"σlogτ1\" -> 1.477924038063   ,  \"σlogτS\" -> 0.000154723460   ,  \"σlogτN\" -> 0.813062124380   ,  \"σητ1\" -> 0.002554352820   ,  \"σητS \" -> 0.000000285180   ,  \"σητN\" -> 0.000001186922    |>   , \n\"IDS0590_220608_RAW_cal__sam_\" ->   <|    \"ζ\" -> 0.000000000000   ,  \"τ1\" -> 0.000000000000   ,  \"τS\" -> 0.000000000000   ,  \"τN\" -> 0.000000000000   ,  \"τC\" -> 0.000000000000   ,  \"κ0\" -> 0.000000000000   ,  \"mm1\" -> 0.000000000000   ,  \"mm2\" -> 0.000000000000   ,  \"mm3\" -> 0.000000000000   ,  \"T\" -> 1.600000000000   ,  \"B\" -> 2.000000000000   ,  \"θ\" -> 90.000000000000   ,  \"Reoff\" -> 0.000000000000   ,  \"Imoff\" -> 0.000000000000   ,  \"στ1\" -> 0.000000000000   ,  \"στS\" -> 0.000000000000   ,  \"στN\" -> 0.000000000000   ,  \"τ11 \" -> 0.000000000000   ,  \"τ12\" -> 0.000000000000   ,  \"τ22\" -> 0.000000000000   ,  \"τN1\" -> 0.000000000000   ,  \"τN2\" -> 0.000000000000   ,  \"σηlogτ1 \" -> 0.000000000000   ,  \"σηlogτS\" -> 0.000000000000   ,  \"σηlogτN\" -> 0.000000000000   ,  \"σlogτ1\" -> 0.000000000000   ,  \"σlogτS\" -> 0.000000000000   ,  \"σlogτN\" -> 0.000000000000   ,  \"σητ1\" -> 0.000000000000   ,  \"σητS \" -> 0.000000000000   ,  \"σητN\" -> 0.000000000000    |>   , \n\"IDS0591_220608_RAW_cal__ref_\" ->   <|    \"ζ\" -> 0.017496232400   ,  \"τ1\" -> 0.009379616300   ,  \"τS\" -> 0.011529506794   ,  \"τN\" -> 0.000002471799   ,  \"τC\" -> 0.003013860200   ,  \"κ0\" -> 0.000000015619   ,  \"mm1\" -> 0.000041347609   ,  \"mm2\" -> 0.009375196223   ,  \"mm3\" -> 0.014710677438   ,  \"T\" -> 2.300000000000   ,  \"B\" -> 2.000000000000   ,  \"θ\" -> 90.000000000000   ,  \"Reoff\" -> 0.000000000000   ,  \"Imoff\" -> 0.000000000000   ,  \"στ1\" -> 0.011594693378   ,  \"στS\" -> 0.000001156302   ,  \"στN\" -> 0.000001553870   ,  \"τ11 \" -> 0.000000000000   ,  \"τ12\" -> 0.000000000000   ,  \"τ22\" -> 0.000000000000   ,  \"τN1\" -> 0.000000000000   ,  \"τN2\" -> 0.000000000000   ,  \"σηlogτ1 \" -> 0.141137332089   ,  \"σηlogτS\" -> 0.000001654332   ,  \"σηlogτN\" -> 0.134661811699   ,  \"σlogτ1\" -> 1.236158602592   ,  \"σlogτS\" -> 0.000100290701   ,  \"σlogτN\" -> 0.628639383488   ,  \"σητ1\" -> 0.001323814021   ,  \"σητS \" -> 0.000000019074   ,  \"σητN\" -> 0.000000332857    |>   , \n\"IDS0591_220608_RAW_cal__sam_\" ->   <|    \"ζ\" -> 0.000000000000   ,  \"τ1\" -> 0.000000000000   ,  \"τS\" -> 0.000000000000   ,  \"τN\" -> 0.000000000000   ,  \"τC\" -> 0.000000000000   ,  \"κ0\" -> 0.000000000000   ,  \"mm1\" -> 0.000000000000   ,  \"mm2\" -> 0.000000000000   ,  \"mm3\" -> 0.000000000000   ,  \"T\" -> 2.300000000000   ,  \"B\" -> 2.000000000000   ,  \"θ\" -> 90.000000000000   ,  \"Reoff\" -> 0.000000000000   ,  \"Imoff\" -> 0.000000000000   ,  \"στ1\" -> 0.000000000000   ,  \"στS\" -> 0.000000000000   ,  \"στN\" -> 0.000000000000   ,  \"τ11 \" -> 0.000000000000   ,  \"τ12\" -> 0.000000000000   ,  \"τ22\" -> 0.000000000000   ,  \"τN1\" -> 0.000000000000   ,  \"τN2\" -> 0.000000000000   ,  \"σηlogτ1 \" -> 0.000000000000   ,  \"σηlogτS\" -> 0.000000000000   ,  \"σηlogτN\" -> 0.000000000000   ,  \"σlogτ1\" -> 0.000000000000   ,  \"σlogτS\" -> 0.000000000000   ,  \"σlogτN\" -> 0.000000000000   ,  \"σητ1\" -> 0.000000000000   ,  \"σητS \" -> 0.000000000000   ,  \"σητN\" -> 0.000000000000    |>   , \n\"IDS0592_220608_RAW_cal__ref_\" ->   <|    \"ζ\" -> 0.019029594007   ,  \"τ1\" -> 0.017581938574   ,  \"τS\" -> 0.009721936381   ,  \"τN\" -> 0.000001128241   ,  \"τC\" -> 0.002339976361   ,  \"κ0\" -> 0.000000022398   ,  \"mm1\" -> 0.000035450791   ,  \"mm2\" -> 0.012208855820   ,  \"mm3\" -> 0.017585698918   ,  \"T\" -> 3.100000000000   ,  \"B\" -> 2.000000000000   ,  \"θ\" -> 90.000000000000   ,  \"Reoff\" -> 0.000000000000   ,  \"Imoff\" -> 0.000000000000   ,  \"στ1\" -> 0.049820756354   ,  \"στS\" -> 0.000000710276   ,  \"στN\" -> 0.000002087356   ,  \"τ11 \" -> 0.000000000000   ,  \"τ12\" -> 0.000000000000   ,  \"τ22\" -> 0.000000000000   ,  \"τN1\" -> 0.000000000000   ,  \"τN2\" -> 0.000000000000   ,  \"σηlogτ1 \" -> 0.093372347104   ,  \"σηlogτS\" -> 0.000000231794   ,  \"σηlogτN\" -> 0.124583503268   ,  \"σlogτ1\" -> 2.833632716014   ,  \"σlogτS\" -> 0.000073059076   ,  \"σlogτN\" -> 1.850098255960   ,  \"σητ1\" -> 0.001641666871   ,  \"σητS \" -> 0.000000002253   ,  \"σητN\" -> 0.000000140560    |>   , \n\"IDS0592_220608_RAW_cal__sam_\" ->   <|    \"ζ\" -> 0.000000000000   ,  \"τ1\" -> 0.000000000000   ,  \"τS\" -> 0.000000000000   ,  \"τN\" -> 0.000000000000   ,  \"τC\" -> 0.000000000000   ,  \"κ0\" -> 0.000000000000   ,  \"mm1\" -> 0.000000000000   ,  \"mm2\" -> 0.000000000000   ,  \"mm3\" -> 0.000000000000   ,  \"T\" -> 3.100000000000   ,  \"B\" -> 2.000000000000   ,  \"θ\" -> 90.000000000000   ,  \"Reoff\" -> 0.000000000000   ,  \"Imoff\" -> 0.000000000000   ,  \"στ1\" -> 0.000000000000   ,  \"στS\" -> 0.000000000000   ,  \"στN\" -> 0.000000000000   ,  \"τ11 \" -> 0.000000000000   ,  \"τ12\" -> 0.000000000000   ,  \"τ22\" -> 0.000000000000   ,  \"τN1\" -> 0.000000000000   ,  \"τN2\" -> 0.000000000000   ,  \"σηlogτ1 \" -> 0.000000000000   ,  \"σηlogτS\" -> 0.000000000000   ,  \"σηlogτN\" -> 0.000000000000   ,  \"σlogτ1\" -> 0.000000000000   ,  \"σlogτS\" -> 0.000000000000   ,  \"σlogτN\" -> 0.000000000000   ,  \"σητ1\" -> 0.000000000000   ,  \"σητS \" -> 0.000000000000   ,  \"σητN\" -> 0.000000000000    |>   , \n\"IDS0593_220608_RAW_cal__ref_\" ->   <|    \"ζ\" -> 0.021294906614   ,  \"τ1\" -> 0.016155792293   ,  \"τS\" -> 0.006010538470   ,  \"τN\" -> 0.000000265204   ,  \"τC\" -> 0.001740380936   ,  \"κ0\" -> 0.000000055295   ,  \"mm1\" -> 0.000028374877   ,  \"mm2\" -> 0.007850282636   ,  \"mm3\" -> 0.016156318893   ,  \"T\" -> 5.700000000000   ,  \"B\" -> 2.000000000000   ,  \"θ\" -> 90.000000000000   ,  \"Reoff\" -> 0.000000000000   ,  \"Imoff\" -> 0.000000000000   ,  \"στ1\" -> 0.179781175728   ,  \"στS\" -> 0.000000482130   ,  \"στN\" -> 0.000002158391   ,  \"τ11 \" -> 0.000000000000   ,  \"τ12\" -> 0.000000000000   , 
